vi "Stop OpenCLV.vi"(8 "Error In":errorcluster) -> (0 "Error Out":errorcluster)   [LabVIEW 2012]
doc: "Cleans up all OpenCLV devices, memory, kernels, programs, and closes the FFT library. \n\nThis should be the very last OpenCLV VI called with the exception of <b>View Log</b>."
uses:
  Non-User VIs/Buffers/Buffer_states.ctl
  OpenCLV x64.lvlib
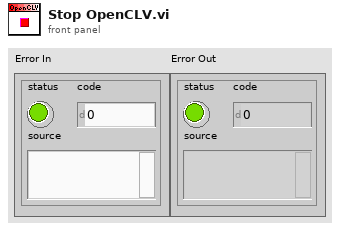
[diagram p1: front panel]
types:
  T1 = typedef "OpenCLV x64.lvlib/Buffer_states.ctl" = enum16{"Purge", "Remove", "Add"}
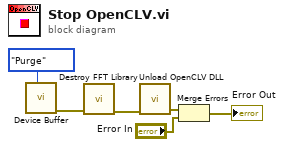
[diagram p0: block diagram]
diagram:
  n1 = call "Device Buffer.vi"("States"=Buffer_states."Purge") -> ("Error Out"=w5:errorcluster)  [unwired: 9 in, 1 out]
  n2 = call "Destroy FFT Library.vi"("Error In"=w5) -> ("Error Out"=w4:errorcluster)  [unwired: 10 in]
  n3 = call "Unload OpenCLV DLL.vi"("Error In"=w4) -> ("Error Out"=w3:errorcluster)  [unwired: 10 in]
  n4 = Merge Errors(w3, "Error In") -> (→"Error Out":errorcluster)
